vi "10-Tap 8-Bit Camera with DRAM (Host) - control.vi"() -> ()   [LabVIEW 2018]
doc: "This is the host VI for the 10-Tap 8-Bit Camera with DRAM example. This example demonstrates how to acquire images from a 10-tap, 8-bit, extended configuration, Camera Link camera and display the images on the host. This example supports area scan and line scan cameras for both continuous and finite acquisitions.\n\nThis example also demonstrates the use of DRAM as a frame buffer for very high speed acquisitions. Data packing and flow-control are also employed to maximize use of the available DRAM and FIFOs in terms of both memory space and performance.\n\nAdditionally, the example demonstrates the serial server, which allows third-party camera configuration utilities to communicate with the camera using the Camera Link serial interface while this VI is running."
uses:
  <vilib>/userdefined/High Color/nirio_resource_hc.ctl
  <vilib>/Platform/TimedLoop/XDataNode/timing_clust.ctl
  <vilib>/Platform/TimedLoop/XDataNode/nitl_modes.ctl
  <vilib>/Platform/TimedLoop/XDataNode/wakeup.ctl
  <vilib>/DAQmx/write.llb/DAQmx Write (Analog DBL 1Chan 1Samp).vi
  <vilib>/FPGAPlugInAG/PCIe-1473R/niLvFpga_Open_PCIe-1473R.vi
  <vilib>/rvi/interface/common/dynamic/niFpgaDynamicAddResources.vi
  <vilib>/FPGAPlugInAG/Dynamic/niLvFpga_Reset_Dynamic.vi
  <userlib>/DAQNavi Polymorphic VI/create/DAQNavi Create Channel(CI-UpDown Count Value).vi
  <vilib>/Utility/error.llb/Error Cluster From Error Code.vi
  <vilib>/rvi/errors/niLvFpgaAdjustHostInterfaceError.vi
  <vilib>/FPGAPlugInAG/Dynamic/niLvFpga_Run_Dynamic.vi
  <vilib>/rvi/interface/common/niFpgaWaitOnOcc.vi
  <userlib>/DAQNavi Polymorphic VI/read/DAQNavi Read (Counter Count Value 1Chan 1Samp).vi
  <vilib>/DAQmx/miscellaneous.llb/DAQmx Fill In Error Info.vi
  <vilib>/FPGAPlugInAG/Dynamic/niLvFpga_Close_Dynamic.vi
  <vilib>/platform/TimedLoop/XDataNode/XDataNode.xnode
  <vilib>/rvi/interface/nirviOpenFPGA/nirviOpenFPGA.xnode
  FPGA Bitfiles/10-Tap8-bitCamer_FPGATarget_10-Tap8-bitCamer_C490DC32.lvbitx
  <vilib>/rvi/interface/nirviMethod/nirviMethod.xnode
  <vilib>/rvi/interface/nirviReadWriteControl/nirviReadWriteControl.xnode
  <vilib>/rvi/interface/nirviCloseFPGA/nirviCloseFPGA.xnode
  <vilib>/rvi/interface/Simulation/niFpgaSimulationCallBeginRW.vi
  <vilib>/rvi/errors/niLvFpgaMergeErrorWithErrorCode.vi
  NiFpgaLv.dll
  <vilib>/FPGAPlugInAG/Dynamic/niLvFpga_ConfigureFifo_Dynamic.vi
  <vilib>/FPGAPlugInAG/Dynamic/niLvFpga_StartFifo_Dynamic.vi
  <vilib>/FPGAPlugInAG/Dynamic/niLvFpga_ReadFifo_Dynamic.vi
  <vilib>/Platform/TimedLoop/XDataNode/XDNodeRunTimeDep.lvlib
  <resource>/objmgr/ni.dex.rc
  MPC_dll_4_vs17_cv3_4/x64/Release/MPC_dll_4_vs17_cv3_4.dll
  fish tracking dll vc17 opencv3_4/x64/Release/fish tracking dll vc17 opencv3_4.dll
panel:
  in  "Templates size":i32=70
  in  "display":bool=TRUE
  out "Image":T1(plugin-control)
  in  "reset 2":bool
  in  "reset frame":bool
  in  "reset position":bool
  out "max load a frame":dbl
  out "max load a position":dbl
  out "# elements in queue":i32
  out "element":dbl[](array[numeric])
  in  "start sending":bool
  in  "Target IP Address":string="192.168.1.19"
  out "connected":bool
  in  "Acquire":bool
  in  "Frames To Acquire":u32 caption="Frames To Acquire\n(0 = infinite)"
  in  "Templates Path":path=path "F:/TrackingUsingOpenCV3_with_bkg_subtr_and_pred_and_temp_matching_nodisplay/templates"
  out "max distance 2":i32
  out "out of FOV 2":i32
  in  "count":bool
  in  "shift_head2yolk":i32=22
  out "max distance":i32
  out "out of FOV":i32
  out "Stage Position Y":i32=520
  out "Stage Position X":i32=520
  out "#timeout3":i32
  out "#timeout1":i32
  out "max time4 image loading":dbl
  out "max time3 total":dbl
  out "max time2 detection":dbl
  out "max time1 detection+command":dbl
  out "time loading a frame":dbl
  in  "gammaY":dbl=0.3 format="%#_13g"
  in  "gammaX":dbl=0.3 format="%#_13g"
  in  "predict length":i32=6
  in  "length of fish_history":i32=3
  in  "m(length of kernel)":i32=30
  out "Heading":cluster{dbl, dbl}
  in  "length_fish":i32=115
  in  "width_fish":i32=23
  out "Time out":bool
  out "BKG_Global":T1(plugin-control)
  in  "update ratio":dbl
  in  "tan(theta)":dbl=-0.0165
  in  "pixel/mm":dbl=29.9
  out "process":i32
  in  "Target Y":i32(slide)=180 min=0 max=384 scale=130.0..230.0
  in  "Target X":i32(slide)=180 min=0 max=520 scale=130.0..230.0
  out "y":dbl
  out "x":dbl
  in  "Controller":picture
  out "Y Resolution":i32
  out "X Resolution":i32
  in  "center":bool
  in  "Track":bool
  out "Frame #":i32=72
  out "电压2":dbl
  out "电压1":dbl
  in  "Bkg Image Path":path=path "F:/TrackingUsingOpenCV3_with_bkg_subtr_and_pred_and_temp_matching_nodisplay/fish tracking dll vc17 opencv3_4/bkg_global.png"
  out "fish FOUND":bool
  in  "Object Threshold":i32=84
  in  "shift":i32=14
  in  "ROI_height":i32=110
  in  "ROI_witdth":i32=110
  out "Centroid":cluster{"x":i32, "y":i32}
  out "TimeDelay":dbl
  in  "BinThreshold":i32=90
  in  "DMA Buffer Size\n(In Images)":u32=64 caption="DMA Buffer Size"
  in  "Signal Mapping":T2(ring)=enum."Basler 10-tap"
  out "Acq In Progress":bool
  in  "Line Scan":bool
  in  "Cancel":bool
  out "Acq'd Frame Width":u32
  in  "Stopped":bool
  in  "RIO Device":T3="RIO0"
  out "DMA Write Timeout":bool
  in  "Start Serial Server":bool=TRUE
  out "Frames Acq'd":u32
  out "Acq'd Frame Height":u32
  in  "Stop":bool
  in  "Image Height":u32=360 max=65535
  in  "Image Width":u32=360 max=65535 step=40
  out "Initialized":bool
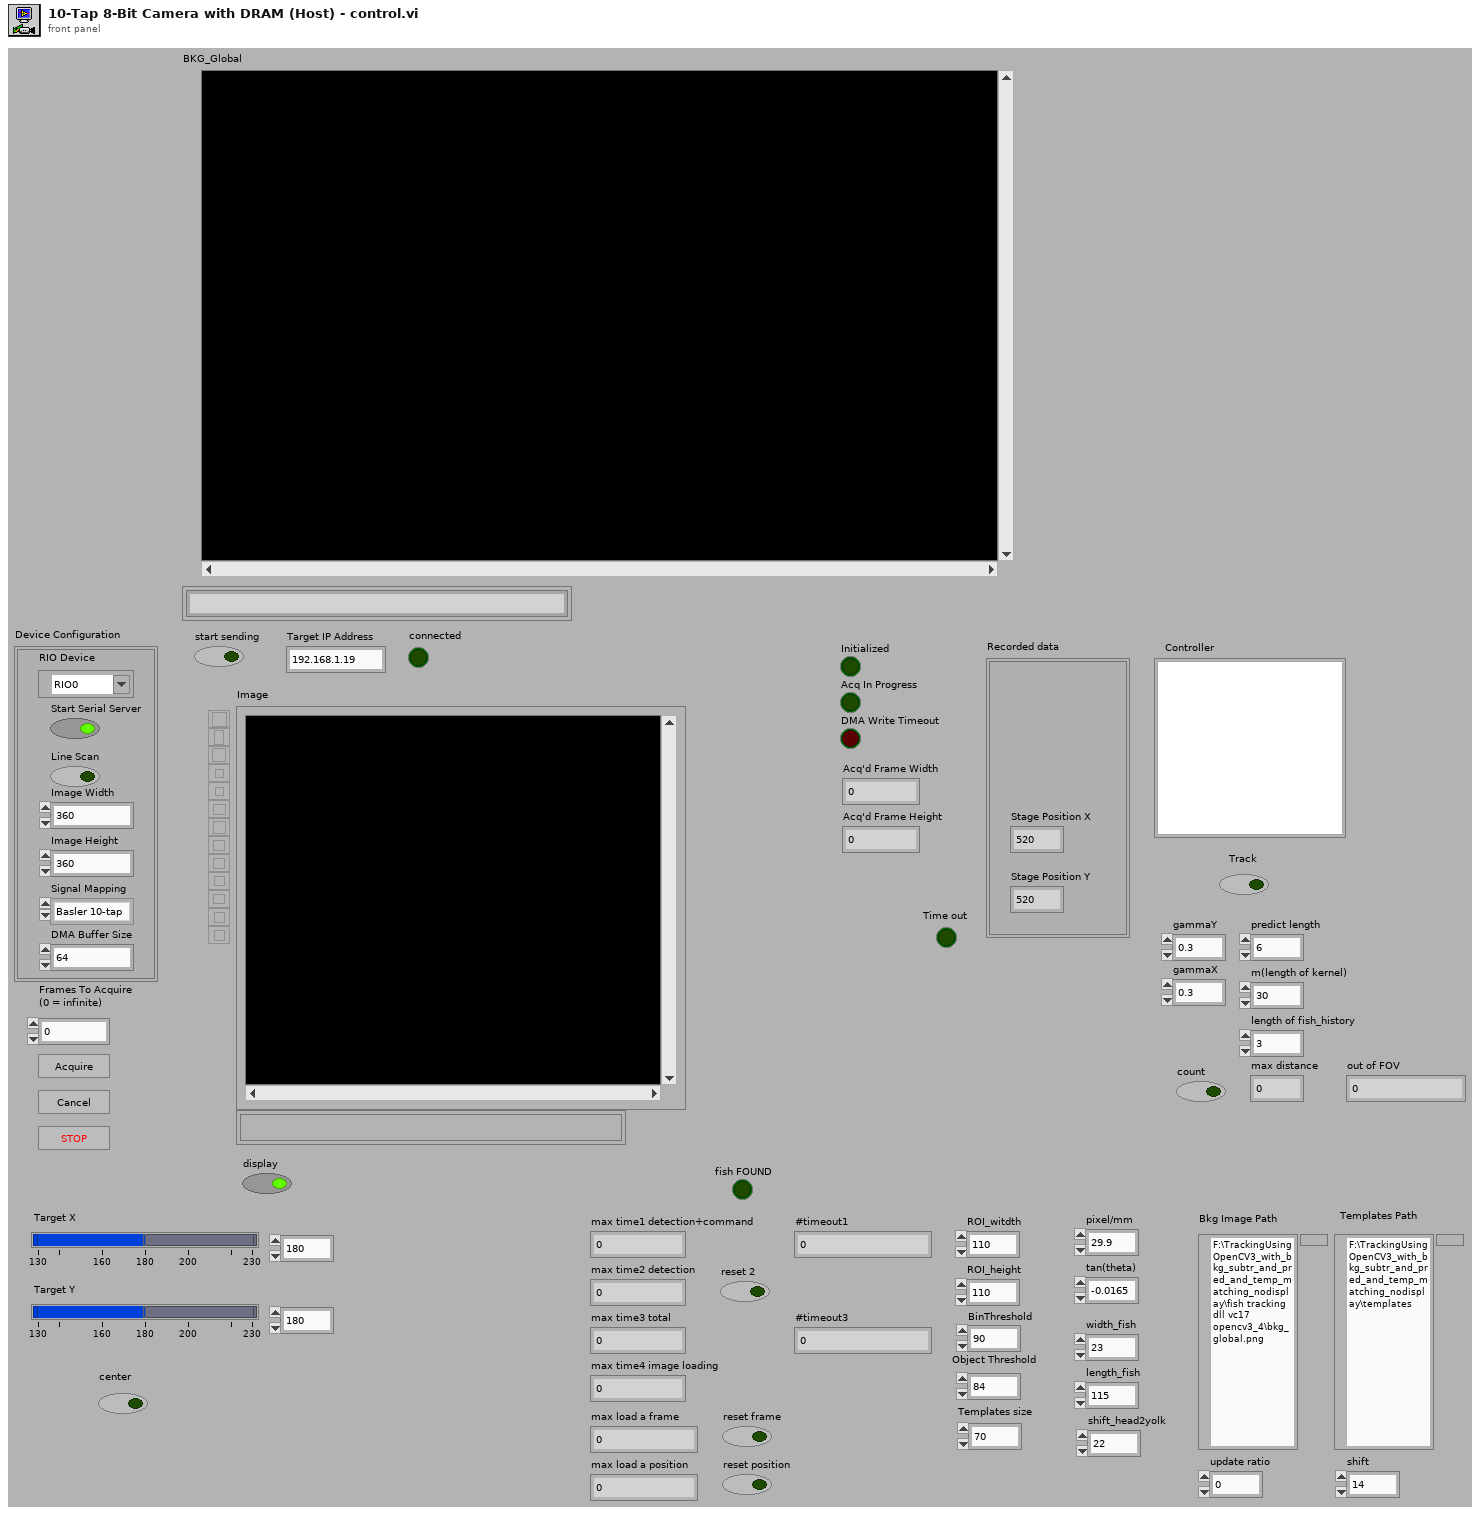
[diagram p1: front panel]
types:
  T1 = typedef "IMAQ Image.ctl" = refnum<image>
  T2 = enum8{"Standard", "Basler 10-tap", "Vosskühler 10-tap"}
  T3 = typedef "nirio_resource_hc.ctl" = tag
  T4 = typedef "Image Type" = u32
  T5 = typedef "XDNodeRunTimeDep.lvlib/timing_clust.ctl" = cluster{"Expected End [f-1]":u64, "Actual End [f-1]":u64, "Finished Late? [f-1]":bool, "Expected End [i-1]":u64, "Actual End [i-1]":u64, "Finished Late? [i-1]":bool, "Expected Start [i]":u64, "Actual Start [i]":u64, "Expected Start [f]":u64, "Actual Start [f]":u64, "Source Name":string, "Structure Name":string, "Period":i64, "Deadline":i64, "Offset":i64, "Start":i64, "Priority":i32, "Timeout":i32, "Mode":T6, "Wakeup Reason":T7, "Error":errorcluster, "Source Type":string, "Secondary Source Type":string, "Global End Time":u64, "Global Start Time":u64, "Frame Duration":u64, "Iteration Duration":u64, "Assigned CPU":i32, "I/O Scan Engine Mode":u32}
  T6 = typedef "XDNodeRunTimeDep.lvlib/nitl_modes.ctl" = enum32{"No Change", "Process missed periods, maintain original phase", "Discard missed periods, maintain original phase", "Process missed periods, ignore original phase", "Discard missed periods, ignore original phase"}
  T7 = typedef "XDNodeRunTimeDep.lvlib/wakeup.ctl" = enum32{"Normal", "Aborted", "Asynchronous wakeup", "Timing source error", "Timed loop error", "Timeout"}
  T8 = enum16{"big-endian, network order", "native, host order", "little-endian"}
  T9 = enum32{"Map Pixel Pointer", "Unmap Pixel Pointer", "Get Pixels Infos"}
  T10 = typedef "LVPoint32TypeDef.ctl" = cluster{"Horizontal":i32, "Vertical":i32}
  T11 = typedef "LVPositionTypeDef.ctl" = cluster{"Left":i32, "Top":i32}
  T12 = typedef "LVBoundsTypeDef.ctl" = cluster{"Width":u32, "Height":u32}
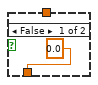
[diagram p6: hidden frame]
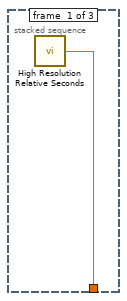
[diagram p7: hidden frame]
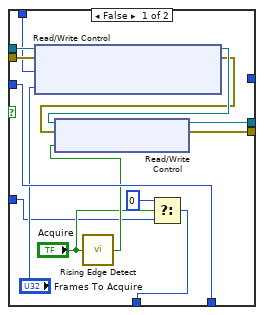
[diagram p8: hidden frame]
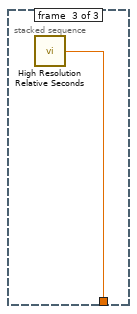
[diagram p9: hidden frame]
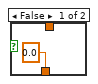
[diagram p10: hidden frame]
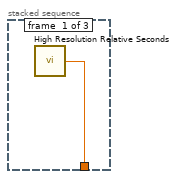
[diagram p11: hidden frame]
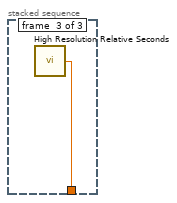
[diagram p12: hidden frame]
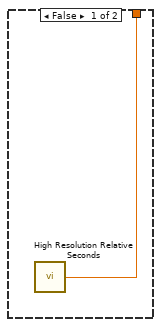
[diagram p18: hidden frame]
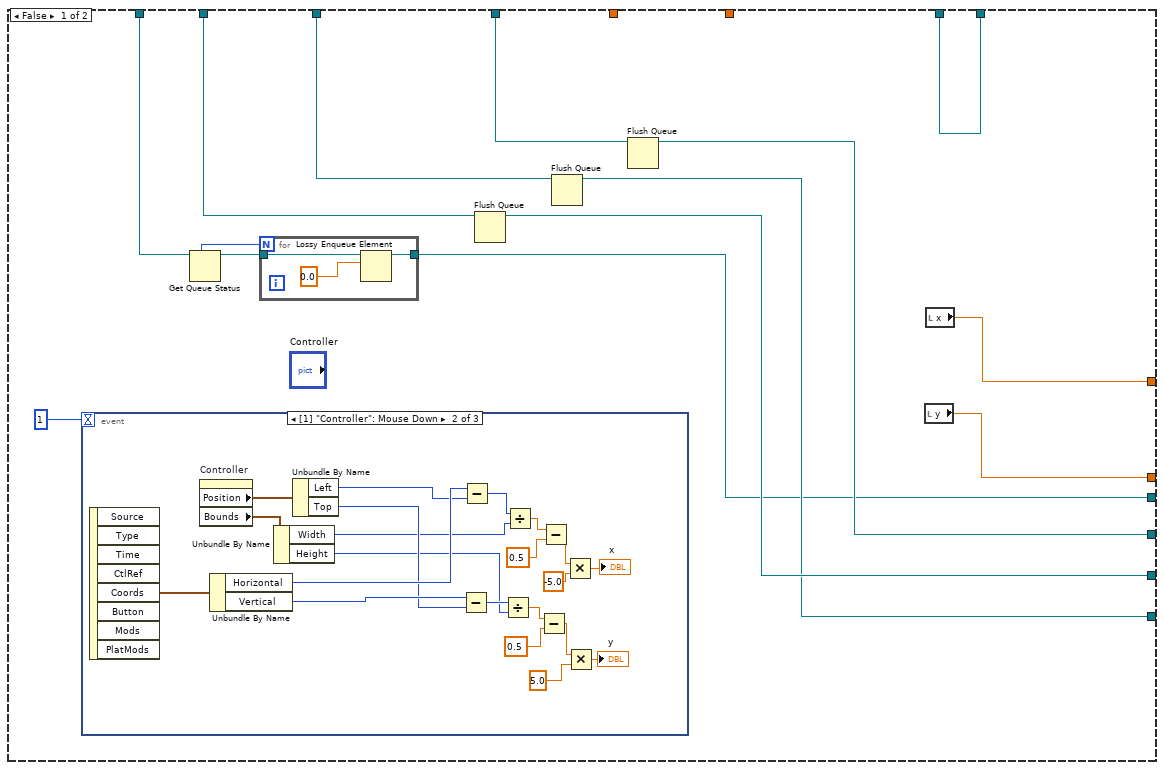
[diagram p20: hidden frame]
diagram:
  w33 = 72 ("n_templates")
  w35 = 0
  w56 = 2
  w50 = 0
  w57 = 0.0
  w82 = T4 0 items=["Grayscale (U8)", "Grayscale (I16)", "Grayscale (SGL)", "Complex (CSG)", "RGB (U32)", "HSL (U32)", "RGB (U64)", "Grayscale (U16)"] ("Image Type")
  w96 = refnum<k21> "Stage_Y"  # DAQmx任务名
  w97 = refnum<k21> "Stage_X"  # DAQmx任务名
  w99 = T4 0 items=["Grayscale (U8)", "Grayscale (I16)", "Grayscale (SGL)", "Complex (CSG)", "RGB (U32)", "HSL (U32)", "RGB (U64)", "Grayscale (U16)"] ("Image Type")
  w105 = u32 8  # Pixels per DMA word
  w139 = T4 0 items=["Grayscale (U8)", "Grayscale (I16)", "Grayscale (SGL)", "Complex (CSG)", "RGB (U32)", "HSL (U32)", "RGB (U64)", "Grayscale (U16)"] ("Image Type")
  # "If your camera outputs active-low enable\nsignals or does not use DVAL then you \ncan change the configuration here."
  # "Configure the DMA FIFO memory buffer to be\nlarge enough for several frames. This provides\nbuffering to help deal with system latencies."
  # "Start running\nthe FPGA VI."
  # "Reset FPGA to clear\nany current state."
  # "Read the specified image\nwidth and height. In this\nexample, these must be set\nbefore starting the VI."
  # "Merge any errors.\nClean up the image.\nClose the FPGA reference.\nDisplay any errors."
  # "Acquire frames as requested.\nUse the width and height to determine how much data to read from the DMA FIFO.\nConvert the data into a Vision Image for display."
  # "Monitor the acquisition status"
  # "Start the Serial Server to allow serial communication\nwith the camera. This allows third-party camera\nconfiguration utilites to be used."
  # "Create an image of the type to be displayed."
  # "Initialize the acquisition interface on the FPGA.  This will\nwait until a pixel clock is detected from the camera."
  # "Initialize the DMA FIFO for transferring\ndata from FPGA target to the host."
  # "Configure the Camera Link interface.\nThis needs to be done prior to running\nthe FPGA block diagram."
  # "Open a reference to the FPGA bitstream\nand initialize the user interface."
  n1 = flat-sequence {
    tunnel: [w145] -> w132
    tunnel: [w144] -> w143
    frame #0 {
      w148 = u32 0 ("Num Lines Acq'd")
      w147 = FALSE ("stop")
      n2 = local write "DMA Write Timeout"(w147) -> ()
      n3 = local write "Acq'd Frame Width"(w148) -> ()
      n4 = local write "Acq'd Frame Height"(w148) -> ()
      n5 = local write "Stopped"(w147) -> ()
      n6 = local write "Frames Acq'd"(w148) -> ()
      n7 = local write "Initialized"(w147) -> ()
      n8 = xnode "打开FPGA VI引用句柄"("resource name"="RIO Device") -> ("FPGA VI Reference Out"=w145:refnum<k20>, "error out"=w144:errorcluster)  [unwired: 1 in]
    }
  }
  n9 = xnode "Invoke Method"("FPGA VI Reference In"=w132, "error in"=w143) -> ("FPGA VI Reference Out"=w122:refnum<k20>, "error out"=w124:errorcluster)
  n10 = xnode "Read/Write Control"("FPGA VI Reference In"=w122, "error in"=w124, "CL Config.FVAL Active High"=TRUE ("IO Module Config.CL FVAL Active High"), "CL Config.LVAL Active High"=TRUE ("IO Module Config.CL LVAL Active High"), "CL Config.DVAL Active High"=TRUE ("IO Module Config.CL DVAL Active High"), "CL Config.Spare Active High"=TRUE ("IO Module Config.CL Spare Active High"), "CL Config.Line Scan"="Line Scan", "Acq Control.Ignore DVAL"=FALSE ("CL Config.Line Scan"), "CL Config.Configuration"=enum8{"Base", "Medium", "Full"}."Full", "CL Config.Signal Mapping"="Signal Mapping") -> ("FPGA VI Reference Out"=w125:refnum<k20>, "error out"=w123:errorcluster)
  n11 = xnode "Invoke Method"("FPGA VI Reference In"=w125, "error in"=w123) -> ("FPGA VI Reference Out"=w102:refnum<k20>, "error out"=w101:errorcluster)  [unwired: 1 in]
  n12 = Multiply(x="Image Height", y="Image Width") -> (x*y=w104:u32)
  n13 = Quotient & Remainder(x=w104, y=w105) -> (floor(x/y)=w103:u32)  [unwired: 1 out]
  n14 = Multiply(x=w103, y="DMA Buffer Size\n(In Images)") -> (x*y=w116:u32)
  n15 = xnode "Invoke Method"("FPGA VI Reference In"=w102, "error in"=w101, "请求的深度"=w116) -> ("FPGA VI Reference Out"=w131:refnum<k20>, "error out"=w130:errorcluster)  [unwired: 1 out]
  n16 = xnode "Invoke Method"("FPGA VI Reference In"=w131, "error in"=w130) -> ("FPGA VI Reference Out"=w117:refnum<k20>, "error out"=w129:errorcluster)
  n17 = xnode "读取/写入控件"("FPGA VI Reference In"=w117, "error in"=w129, "Acq Control.Initialize"=TRUE ("Arm Acquisition")) -> ("FPGA VI Reference Out"=w142:refnum<k20>, "error out"=w141:errorcluster)
  n18 = while {
    tunnel: w142 -> [w156]
    tunnel: w141 -> [w155]
    tunnel: [w154] -> w113
    tunnel: [w158] -> w112
    i -> [w150]
    stop <- w161 stop-if-true
    # "A custom error is generated if the acquisition unit has not become\ninitialized within 2 seconds. This typically occurs when a camera is\nnot connected, is not powered, or is not of the correct type."
    n19 = xnode "读取/写入控件"("FPGA VI Reference In"=w156, "error in"=w155) -> ("FPGA VI Reference Out"=w154:refnum<k20>, "error out"=w153:errorcluster, "Acq Status.Initialized"=w152:bool)
    n20 = Wait (ms)(milliseconds to wait=u32 100) -> ()  [unwired: 1 out]
    n21 = Greater?(x=w150, y=20) -> (0:w151:bool)
    n22 = case shown="True" w151 {
      tunnel: [w163 FALSE] -> w157
      tunnel: w152 -> [w163 _]
      tunnel: w153 -> [w162 w165]
      tunnel: [w162 w167] -> w158
      frame False {
      }
      frame True {
        n23 = Merge Errors(w165, errorcluster {"status"=TRUE, "code"=-8999, "source"="Acquisition Initialization: This error typically occurs when a camera is not properly connected, is not powered, or is not of the correct type."} ("error in")) -> (w167:errorcluster)
      }
    }
    "Initialized" <- w157
    n24 = Unbundle By Name(w158) -> ("status"=w160:bool)
    n25 = Or(x=w160, y=w157) -> (x .or. y?=w161:bool)
  }
  n26 = case shown="True" "Start Serial Server" {
    tunnel: [_ w168] -> w133
    tunnel: w113 -> [_ w169]
    frame False {
    }
    frame True {
      n27 = control-ref of="Stopped"() -> (w170:refnum<vi>)
      n28 = call "SerialServer.vi"("Stop Refnum"=w170, "FPGA VI Reference In"=w169) -> ("FPGA VI Reference Out"=w168:refnum<k20>)  [unwired: 5 in]
    }
  }
  n29 = call "IMAQ Create"("Image Name"="Image", "Image Type"=w139, "error in (no error)"=w112) -> ("New Image"=w109:T1, "error out"=w108:errorcluster)  [unwired: 2 in]
  n30 = Concatenate Strings("//" ("reader url"), "Target IP Address") -> (w17:string)
  n31 = Concatenate Strings(w17, "/reader1" ("reader url")) -> (w15:string)
  n32 = Create Network Stream Writer Endpoint(7:70, 9:0.0, 10:w15, 11:"writer") -> (0:w20:errorcluster, 3:w22:refnum<k21>)  [unwired: 3 in]
  n33 = property class="Network Stream Endpoint"(reference=w22, error in=w20) -> (reference out=w9:refnum<k21>, error out=w8:errorcluster, "Connected"=→"connected":bool)
  n34 = Add(x="length of fish_history", y=1) -> (x+y=w52:i32)
  n35 = Initialize Array(0.0, 7) -> (w12:dbl[])
  n36 = Obtain Queue(max queue size (-1, unlimited)=3, name (unnamed)="tracking result" ("Image Name"), element data type=w12) -> (queue out=w10:refnum<queue>)  [unwired: 2 in, 2 out]
  n37 = Multiply(x=w56, y=w52) -> (x*y=w49:i32)
  n38 = To Unsigned Byte Integer(number=w35) -> (unsigned 8bit integer=w36:u8)
  n39 = Initialize Array(w36, w35, w35, w35) -> (w34:u8[][][])
  n40 = node-c288() -> (w7:T5)  [unwired: 4 in]
  n41 = for {
    N: w33 -> [_]
    shift-right: [w172] -> w32
    shift-left: w34 -> [w173]
    i -> [w171]
    w177 = T4 0 items=["Grayscale (U8)", "Grayscale (I16)", "Grayscale (SGL)", "Complex (CSG)", "RGB (U32)", "HSL (U32)", "RGB (U64)", "Grayscale (U16)"] ("Image Type")
    n42 = Number To Decimal String(number=w171) -> (decimal integer string=w181:string)  [unwired: 1 in]
    n43 = Concatenate Strings(w181, ".jpg") -> (w180:string)
    n44 = Build Path(base path="Templates Path", name or relative path=w180) -> (appended path=w179:path)
    n45 = call "IMAQ Create"("Image Name"="Temp", "Image Type"=w177) -> ("New Image"=w176:T1)  [unwired: 3 in, 1 out]
    n46 = call "IMAQ ReadFile"("File Path"=w179, "Image"=w176) -> ("Image Out"=w175:T1)  [unwired: 5 in, 4 out]
    n47 = call "IMAQ ImageToArray"("Image"=w175) -> ("Image Pixels (U8)"=w174:u8[][])  [unwired: 3 in, 4 out]
    n48 = Insert Into Array(array=w173, index (dim 0)=w171, new element=w174) -> (w172:u8[][][])  [unwired: 2 in]
  }
  n49 = Add(x="m(length of kernel)", y=1) -> (x+y=w37:i32)
  n50 = timed-loop {
    tunnel: w10 -> [w190]
    tunnel: w9 -> [w189]
    tunnel: w8 -> [w188]
    tunnel: [w187] -> w3
    tunnel: [w186] -> w2
    tunnel: [w185] -> w1
    timing: w7 -> [_]
    timing-out: [_] -> w6
    stop <- w184 stop-if-true
    n51 = node-c288() -> ()  [unwired: 1 in, 1 out]
    n52 = case shown="True" "start sending" {
      tunnel: w189 -> [w195 w208]
      tunnel: w188 -> [w194 w207]
      tunnel: w190 -> [w196 w198]
      tunnel: [w196 w206] -> w187
      tunnel: [w195 w201] -> w186
      tunnel: [w194 w200] -> w185
      frame False {
      }
      frame True {
        w202 = 0
        n53 = Get Queue Status(queue=w198) -> (queue out=w199:refnum<queue>, # elements in queue=w197:i32)  [unwired: 2 in, 6 out]
        n54 = disable-structure shown="Disabled" {
          disable-tunnel: w197 -> [w209 _]
          frame Disabled {
            "# elements in queue" <- w209
          }
          frame Enabled {
          }
        }
        n55 = Dequeue Element(queue=w199) -> (queue out=w206:refnum<queue>, element=w205:dbl[])  [unwired: 2 in, 2 out]
        n56 = disable-structure shown="Disabled" {
          disable-tunnel: w205 -> [w210 _]
          frame Disabled {
            "element" <- w210
          }
          frame Enabled {
          }
        }
        n57 = shared-variable-write(w208, w207, w205, w202) -> (w204:refnum<k21>, w203:errorcluster)  [unwired: 1 out]
        n58 = Flush Stream(8:w203, 9:w202, 11:w204) -> (0:w200:errorcluster, 3:w201:refnum<k21>)  [unwired: 1 in, 1 out]
      }
    }
    n59 = local read "Stop"() -> (w184:bool)
    n60 = node-c288() -> ()  [unwired: 1 in, 1 out]
  }
  n61 = Multiply(x=w56, y=w37) -> (x*y=w55:i32)
  n62 = Obtain Queue(max queue size (-1, unlimited)=w55, name (unnamed)="command_history", element data type=w57) -> (queue out=w59:refnum<queue>)  [unwired: 2 in, 2 out]
  n63 = Obtain Queue(max queue size (-1, unlimited)=w49, name (unnamed)="stage_position_history", element data type=w50) -> (queue out=w48:refnum<queue>)  [unwired: 2 in, 2 out]
  n64 = Obtain Queue(max queue size (-1, unlimited)=w49, name (unnamed)="fish_tr_history", element data type=w50) -> (queue out=w61:refnum<queue>)  [unwired: 2 in, 2 out]
  n65 = Obtain Queue(max queue size (-1, unlimited)=w49, name (unnamed)="fish_heading_history", element data type=w57) -> (queue out=w60:refnum<queue>)  [unwired: 2 in, 2 out]
  n66 = for "For循环" {
    N: w55 -> [_]
    tunnel: w59 -> [w213]
    tunnel: [w212] -> w58
    n67 = Lossy Enqueue Element(queue=w213, element=0.0) -> (queue out=w212:refnum<queue>)  [unwired: 1 in, 3 out]
  }
  n68 = call-poly <userlib>:"DAQNavi Create Channel.vi"("physical channels"="PCI-1784,BID#1/cntr0" ("Image Name"), "signal counting type"="AbPhaseX4" ("Image Name"), "initial value"="0" ("Image Name")) -> ("task out"=w76:i32)  [unwired: 11 in, 1 out]
  n69 = call-poly <userlib>:"DAQNavi Create Channel.vi"("physical channels"="PCI-1784,BID#1/cntr1" ("Image Name"), "signal counting type"="AbPhaseX4" ("Image Name"), "initial value"="0" ("Image Name")) -> ("task out"=w75:i32)  [unwired: 11 in, 1 out]
  n70 = call "IMAQ Create"("Image Name"="BkgImageOpenCV", "Image Type"=w82) -> ("New Image"=w84:T1)  [unwired: 3 in, 1 out]
  n71 = node-c288() -> (w27:T5)  [unwired: 4 in]
  n72 = call <userlib>:"DAQNavi Start Task.vi"("task in"=w76) -> ("task out"=w72:i32)  [unwired: 9 in, 1 out]
  n73 = call <userlib>:"DAQNavi Start Task.vi"("task in"=w75) -> ("task out"=w71:i32)  [unwired: 9 in, 1 out]
  n74 = call "IMAQ Create"("Image Name"="DstImageOpenCV", "Image Type"=w99) -> ("New Image"=w98:T1)  [unwired: 3 in, 1 out]
  n75 = call "IMAQ ReadFile"("File Path"="Bkg Image Path", "Image"=w84) -> ("Image Out"=w81:T1)  [unwired: 5 in, 4 out]
  n76 = while {
    tunnel: w113 -> [w224]
    tunnel: [w227] -> w126
    stop <- w226 stop-if-true
    w217 = u32 10  # Pixels per clock
    # "Update status indicators"
    n77 = Wait Until Next ms Multiple(millisecond multiple=u32 100) -> ()  [unwired: 1 out]
    n78 = xnode "Read/Write Control"("FPGA VI Reference In"=w224) -> ("error out"=w223:errorcluster, "Acq Status.Lines Per Frame"=→"Acq'd Frame Height":u32, "Acq Status.Frames Acq'd"=→"Frames Acq'd":u32, "Acq Status.Clocks Per Line"=w218:u32, "Acq Status.Acq In Progress"=→"Acq In Progress":bool, "Acq Status.DMA Write Timeout"=w215:bool)  [unwired: 1 in, 1 out]
    "DMA Write Timeout" <- w215
    n79 = Multiply(x=w218, y=w217) -> (x*y=→"Acq'd Frame Width":u32)
    n80 = local read "Stopped"() -> (w214:bool)
    n81 = Compound Arithmetic op=AND(w215, invert w214) -> (w216:bool)
    n82 = case shown="True" w216 {
      tunnel: w223 -> [w232 _]
      tunnel: [w232 errorcluster {"status"=TRUE, "code"=-8999, "source"="DMA Write Timeout: The write operation to the DMA FIFO on the FPGA timed out. This can be caused by the DMA FIFO not being started or the DMA FIFO overflowing. Make sure that Start is being called on the DMA FIFO. Also make sure that the host application is reading from the DMA FIFO fast enough to prevent it from overflowing."} ("error out")] -> w227
      frame False {
      }
      frame True {
      }
    }
    n83 = flat-sequence {
      tunnel: w227 -> [w231]
      tunnel: [w229] -> w226
      frame #0 {
        n84 = Unbundle By Name(w231) -> ("status"=w230:bool)
        n85 = Or(x=w230, y="Stopped") -> (x .or. y?=w229:bool)
        n86 = local write "Stopped"(w229) -> ()
      }
    }
  }
  n87 = node-c288(w6) -> ()  [unwired: 1 out]
  n88 = Release Queue(queue=w3) -> ()  [unwired: 2 in, 3 out]
  n89 = Flush Stream(8:w1, 11:w2) -> (0:w4:errorcluster, 3:w5:refnum<k21>)  [unwired: 2 in, 1 out]
  n90 = Destroy Stream Endpoint(8:w4, 11:w5) -> ()  [unwired: 1 out]
  n91 = Open/Create/Replace File(file path (use dialog)=path "E:/Time.txt" ("Folder"), operation (0:open)=4) -> (refnum out=w41:refnum<file>)  [unwired: 4 in, 2 out]
  n92 = call <vilib>:"DAQmx Start Task.vi"("task/channels in"=w96) -> ("task out"=w94:refnum<k21>)  [unwired: 13 in, 1 out]
  n93 = call <vilib>:"DAQmx Start Task.vi"("task/channels in"=w97) -> ("task out"=w95:refnum<k21>)  [unwired: 13 in, 1 out]
  n94 = timed-loop {
    tunnel: w113 -> [w351]
    tunnel: w108 -> [w350]
    tunnel: w103 -> [w247]
    tunnel: "Image Height" -> [w246]
    tunnel: "Image Width" -> [w355]
    tunnel: w109 -> [w354]
    tunnel: [w236] -> w127
    tunnel: [w353] -> w138
    tunnel: [w352] -> w135
    tunnel: w98 -> [w349]
    tunnel: w95 -> [w348]
    tunnel: w94 -> [w347]
    tunnel: [w346] -> w93
    tunnel: [w345] -> w92
    tunnel: w81 -> [w344]
    tunnel: w72 -> [w337]
    tunnel: w71 -> [w336]
    tunnel: [w335] -> w68
    tunnel: [w334] -> w67
    shift-right: [w340] -> _
    shift-left: u32 0 -> [w341]
    shift-right: [w338] -> _
    shift-left: cluster{"y":i32, "x":i32} {"y"=0, "x"=0} ("Centroid") -> [w339]
    tunnel: w58 -> [w333]
    tunnel: w61 -> [w332]
    tunnel: w60 -> [w331]
    tunnel: w48 -> [w330]
    tunnel: [w329] -> w47
    tunnel: [w328] -> w46
    tunnel: [w327] -> w45
    tunnel: [w326] -> w44
    tunnel: w41 -> [w324]
    tunnel: [w323] -> w40
    shift-right: [w322] -> _
    shift-left: _ -> [w321]
    tunnel: w33 -> [w320]
    tunnel: w32 -> [w319]
    tunnel: w10 -> [w318]
    timing: w27 -> [_]
    timing-out: [_] -> w26
    border: u32 0 -> [_]
    i -> [w325]
    stop <- w342 stop-if-true
    # "Read one frame\nfrom DMA FIFO"
    # "If we're in an acquisition, wait until\nwe have at least one frame to read."
    n95 = node-c288() -> ()  [unwired: 1 in, 1 out]
    n96 = stacked-sequence {
      tunnel: [_ w366 _] -> w353
      tunnel: w351 -> [_ w365 _]
      tunnel: w350 -> [_ w364 _]
      tunnel: [_ w363 _] -> w236
      tunnel: [_ w362 _] -> w317
      tunnel: w247 -> [_ w361 _]
      tunnel: w246 -> [_ w360 _]
      tunnel: [w359 _ _] -> w244
      tunnel: [_ _ w414] -> w245
      frame #0 {
        n97 = call <vilib>:"High Resolution Relative Seconds.vi"() -> ("relative seconds"=w359:dbl)
      }
      frame #1 {
        n98 = while {
          tunnel: [w372] -> w362
          tunnel: w361 -> [w369]
          shift-right: [w380] -> w366
          shift-left: w365 -> [w379]
          shift-right: [w373] -> w363
          shift-left: w364 -> [w378]
          tunnel: w360 -> [w367]
          stop <- w368 stop-if-true
          n99 = feedback #1() -> (w374:u32)
          n100 = while {
            tunnel: w379 -> [w410]
            tunnel: w378 -> [w409]
            tunnel: [w407] -> w377
            tunnel: [w408] -> w376
            tunnel: w374 -> [w413]
            tunnel: [w411] -> w370
            stop <- w412 stop-if-true
            n101 = xnode "Read/Write Control"("FPGA VI Reference In"=w410, "error in"=w409, "Acq Control.Cancel Acq"="Cancel") -> ("FPGA VI Reference Out"=w408:refnum<k20>, "error out"=w407:errorcluster, "Acq Status.Acq In Progress"=w406:bool, "Acq Status.Frames Acq'd"=w405:u32)
            n102 = Greater?(x=w405, y=w413) -> (0:w411:bool)
            n103 = Compound Arithmetic op=OR(invert w406, w411) -> (w412:bool)
          }
          n104 = case shown="True" w370 {
            tunnel: w369 -> [w392 w403]
            tunnel: [w387 w402] -> w380
            tunnel: w377 -> [w394 w401]
            tunnel: w376 -> [w393 w400]
            tunnel: [w381 w399] -> w375
            tunnel: w374 -> [w382 w398]
            tunnel: [w386 w397] -> w373
            tunnel: [_ w396] -> w372
            tunnel: [w392 w395] -> w371
            tunnel: w367 -> [w391 _]
            frame False {
              n105 = xnode "Read/Write Control"("FPGA VI Reference In"=w393, "error in"=w394, "Acq Control.Line Scan Height"=w391, "Acq Control.Frames To Acq"="Frames To Acquire") -> ("FPGA VI Reference Out"=w389:refnum<k20>, "error out"=w388:errorcluster)
              n106 = call "Rising Edge Detect.vi"("Input"="Acquire") -> ("Pulse"=w385:bool)  [unwired: 4 in]
              n107 = xnode "Read/Write Control"("FPGA VI Reference In"=w389, "error in"=w388, "Acq Control.Acquire"=w385) -> ("FPGA VI Reference Out"=w387:refnum<k20>, "error out"=w386:errorcluster)
              n108 = Select(t=u32 0, s="Acquire", f=w382) -> (s? t:f=w381:u32)
            }
            frame True {
              n109 = xnode "Invoke Method"("FPGA VI Reference In"=w400, "error in"=w401, "元素数量"=w403) -> ("FPGA VI Reference Out"=w402:refnum<k20>, "error out"=w397:errorcluster, "数据"=w396:u64[], "剩余元素"=w395:u32)  [unwired: 1 in]
              n110 = Increment(x=w398) -> (x+1=w399:u32)
            }
          }
          n111 = feedback-in #1(w375) -> ()
          n112 = Less?(x=w371, y=w369) -> (x < y?=w368:bool)
        }
      }
      frame #2 {
        n113 = call <vilib>:"High Resolution Relative Seconds.vi"() -> ("relative seconds"=w414:dbl)
      }
    }
    n114 = disable-structure shown="Disabled" {
      disable-tunnel: w325 -> [w356 _]
      frame Disabled {
        "process" <- w356
      }
      frame Enabled {
      }
    }
    n115 = Not(x="reset frame") -> (.not. x?=w235:bool)
    n116 = Boolean To (0,1)(Boolean=w235) -> (0, 1=w240:i16)
    n117 = Subtract(x=w245, y=w244) -> (x-y=w241:dbl)
    n118 = feedback #2(-inf) -> (w243:dbl)
    n119 = Max & Min(x=w241, y=w243) -> (max(x,y)=w238:dbl)  [unwired: 1 out]
    n120 = Multiply(x=w238, y=w240) -> (x*y=w237:dbl)
    n121 = feedback-in #2(w237) -> ()
    n122 = case shown="True" w235 {
      tunnel: w238 -> [_ w358]
      tunnel: [0.0 w358] -> w234
      frame False {
      }
      frame True {
      }
    }
    "max load a frame" <- w234
    n123 = flat-sequence {
      tunnel: w321 -> [w434]
      tunnel: w330 -> [w435]
      tunnel: w331 -> [w436]
      tunnel: w332 -> [w437]
      tunnel: w333 -> [w438]
      tunnel: w336 -> [w432]
      tunnel: w337 -> [w433]
      tunnel: w339 -> [w439]
      tunnel: w341 -> [w440]
      tunnel: w344 -> [w441]
      tunnel: w349 -> [w442]
      tunnel: w317 -> [w443]
      tunnel: w354 -> [w444]
      tunnel: w355 -> [w445]
      tunnel: w246 -> [w446]
      tunnel: [w446] -> w316
      tunnel: [w445] -> w315
      tunnel: [w444] -> w314
      tunnel: [w443] -> w313
      tunnel: [w442] -> w312
      tunnel: [w441] -> w311
      tunnel: [w440] -> w310
      tunnel: [w439] -> w309
      tunnel: [w438] -> w308
      tunnel: [w437] -> w307
      tunnel: [w436] -> w306
      tunnel: [w435] -> w305
      tunnel: [w434] -> w304
      tunnel: [w431] -> w303
      tunnel: [w430] -> w302
      tunnel: [w429] -> w301
      tunnel: [w428] -> w300
      tunnel: w320 -> [w428]
      tunnel: [w427] -> w299
      tunnel: w319 -> [w427]
      tunnel: w318 -> [w426]
      tunnel: [w426] -> w298
      tunnel: [w489] -> w297
      tunnel: [w488] -> w296
      tunnel: [w487] -> w295
      tunnel: [w486] -> w294
      tunnel: [w485] -> w293
      tunnel: [w484] -> w292
      tunnel: [w483] -> w291
      tunnel: [w482] -> w290
      tunnel: [w464] -> w289
      tunnel: [w462] -> w288
      tunnel: [w481] -> w287
      tunnel: [w480] -> w286
      tunnel: [w479] -> w285
      tunnel: [w478] -> w284
      tunnel: [w474] -> w283
      tunnel: [w463] -> w282
      tunnel: w316 -> [w489]
      tunnel: w315 -> [w488]
      tunnel: w314 -> [w487]
      tunnel: w313 -> [w486]
      tunnel: w312 -> [w485]
      tunnel: w311 -> [w484]
      tunnel: w310 -> [w483]
      tunnel: w309 -> [w482]
      tunnel: w308 -> [w481]
      tunnel: w307 -> [w480]
      tunnel: w306 -> [w479]
      tunnel: w305 -> [w478]
      tunnel: w304 -> [w472]
      tunnel: w303 -> [w464]
      tunnel: w302 -> [w463]
      tunnel: w301 -> [w462]
      tunnel: [w461] -> w281
      tunnel: w300 -> [w461]
      tunnel: [w460] -> w280
      tunnel: w299 -> [w460]
      tunnel: [w459] -> w279
      tunnel: w298 -> [w459]
      tunnel: w325 -> [w525]
      tunnel: w324 -> [w524]
      tunnel: [w523] -> w323
      tunnel: w297 -> [w575]
      tunnel: w296 -> [w574]
      tunnel: w295 -> [w573]
      tunnel: w294 -> [w571]
      tunnel: w293 -> [w494]
      tunnel: w292 -> [w545]
      tunnel: w291 -> [w542]
      tunnel: w290 -> [w492]
      tunnel: w289 -> [w518]
      tunnel: w288 -> [w517]
      tunnel: w287 -> [w536]
      tunnel: w286 -> [w535]
      tunnel: w285 -> [w534]
      tunnel: w284 -> [w533]
      tunnel: w283 -> [w521]
      tunnel: [w495] -> w278
      tunnel: [w541] -> w277
      tunnel: [w518] -> w276
      tunnel: [w517] -> w275
      tunnel: [w504] -> w274
      tunnel: [w532] -> w273
      tunnel: [w531] -> w272
      tunnel: [w530] -> w271
      tunnel: [w529] -> w270
      tunnel: [w520] -> w269
      tunnel: [w519] -> w268
      tunnel: w282 -> [w505]
      tunnel: w281 -> [w515]
      tunnel: w280 -> [w513]
      tunnel: w279 -> [w508]
      tunnel: w278 -> [w826]
      tunnel: [w826] -> w267
      tunnel: w277 -> [w825]
      tunnel: [w825] -> w266
      tunnel: w276 -> [w824]
      tunnel: [w824] -> w265
      tunnel: w275 -> [w823]
      tunnel: [w823] -> w264
      tunnel: w274 -> [w822]
      tunnel: [w822] -> w263
      tunnel: w273 -> [w821]
      tunnel: [w821] -> w262
      tunnel: w272 -> [w820]
      tunnel: [w820] -> w261
      tunnel: w271 -> [w819]
      tunnel: [w819] -> w260
      tunnel: w270 -> [w818]
      tunnel: [w818] -> w259
      tunnel: w269 -> [w817]
      tunnel: [w817] -> w258
      tunnel: w268 -> [w816]
      tunnel: [w816] -> w257
      tunnel: w267 -> [w842]
      tunnel: w266 -> [w841]
      tunnel: w265 -> [w840]
      tunnel: w264 -> [w839]
      tunnel: w263 -> [w838]
      tunnel: w262 -> [w837]
      tunnel: w261 -> [w836]
      tunnel: w260 -> [w835]
      tunnel: w259 -> [w834]
      tunnel: [w833] -> w345
      tunnel: [w832] -> w346
      tunnel: w348 -> [w831]
      tunnel: w347 -> [w830]
      tunnel: w258 -> [w829]
      tunnel: w257 -> [w828]
      tunnel: [w842] -> w256
      tunnel: [w841] -> w255
      tunnel: [w840] -> w254
      tunnel: [w839] -> w253
      tunnel: [w838] -> w252
      tunnel: [w837] -> w251
      tunnel: [w836] -> w250
      tunnel: [w835] -> w249
      tunnel: [w834] -> w248
      tunnel: [w844] -> w326
      tunnel: [w845] -> w327
      tunnel: [w846] -> w328
      tunnel: [w847] -> w329
      tunnel: [w848] -> w338
      tunnel: [w849] -> w334
      tunnel: [w850] -> w335
      tunnel: [w851] -> w340
      tunnel: [w852] -> w352
      tunnel: w256 -> [w852]
      tunnel: w255 -> [w851]
      tunnel: w254 -> [w850]
      tunnel: w253 -> [w849]
      tunnel: w252 -> [w848]
      tunnel: w251 -> [w847]
      tunnel: w250 -> [w846]
      tunnel: w249 -> [w845]
      tunnel: w248 -> [w844]
      tunnel: [w843] -> w322
      frame #0 {
        n124 = stacked-sequence {
          tunnel: w433 -> [_ w456 _]
          tunnel: w432 -> [_ w455 _]
          tunnel: [_ w454 _] -> w431
          tunnel: [_ w453 _] -> w430
          tunnel: [_ w452 _] -> w429
          tunnel: [w449 _ _] -> w425
          tunnel: [_ _ w458] -> w424
          frame #0 {
            n125 = call <vilib>:"High Resolution Relative Seconds.vi"() -> ("relative seconds"=w449:dbl)
          }
          frame #1 {
            n126 = call-poly <userlib>:"DAQNavi Read.vi"("task in"=w455) -> ("data"=w451:i32, "task out"=w452:i32)  [unwired: 9 in]
            n127 = call-poly <userlib>:"DAQNavi Read.vi"("task in"=w456) -> ("data"=w457:i32, "task out"=w454:i32)  [unwired: 9 in]
            "Stage Position X" <- w457
            n128 = Negate(x=w451) -> (-x=w450:i32)
            "Stage Position Y" <- w450
            n129 = Bundle("data"=w457, w450) -> (w453:cluster{"data":i32, i32})  [unwired: 1 in]
          }
          frame #2 {
            n130 = call <vilib>:"High Resolution Relative Seconds.vi"() -> ("relative seconds"=w458:dbl)
          }
        }
        n131 = Not(x="reset position") -> (.not. x?=w417:bool)
        n132 = Boolean To (0,1)(Boolean=w417) -> (0, 1=w419:i16)
        n133 = Subtract(x=w424, y=w425) -> (x-y=w421:dbl)
        n134 = feedback #3(-inf) -> (w423:dbl)
        n135 = Max & Min(x=w421, y=w423) -> (max(x,y)=w416:dbl)  [unwired: 1 out]
        n136 = Multiply(x=w416, y=w419) -> (x*y=w418:dbl)
        n137 = feedback-in #3(w418) -> ()
        n138 = case shown="True" w417 {
          tunnel: w416 -> [_ w448]
          tunnel: [0.0 w448] -> w415
          frame False {
          }
          frame True {
          }
        }
        "max load a position" <- w415
      }
      frame #1 {
        n139 = call <vilib>:"High Resolution Relative Seconds.vi"() -> ("relative seconds"=w474:dbl)
        n140 = feedback #4() -> (w475:dbl)  [unwired: 1 in]
        n141 = feedback-in #4(w474) -> ()
        n142 = Subtract(x=w474, y=w475) -> (x-y=w477:dbl)
        n143 = disable-structure shown="Disabled" {
          disable-tunnel: w477 -> [w490 _]
          frame Disabled {
            "TimeDelay" <- w490
          }
          frame Enabled {
          }
        }
        n144 = Greater?(x=w477, y=0.0045) -> (0:w469:bool)
        "Time out" <- w469
        n145 = Subtract(x=w474, y=w472) -> (x-y=w473:dbl)
        n146 = disable-structure shown="Disabled" {
          disable-tunnel: w473 -> [w491 _]
          frame Disabled {
            "time loading a frame" <- w491
          }
          frame Enabled {
          }
        }
        n147 = Select(t=1, s=w469, f=0) -> (s? t:f=w466:i32)
        n148 = feedback #5(0) -> (w467:i32)
        n149 = Add(x=w466, y=w467) -> (x+y=w465:i32)
        "#timeout3" <- w465
        n150 = feedback-in #5(w465) -> ()
      }
      frame #2 {
        w537 = 0.0
        w556 = T9."Map Pixel Pointer" ("Function")
        # "Convert U64 array\nto U8 array"
        # "Convert array to\nimage for display"
        n151 = Add(x=1, y=w542) -> (x+y=w541:u32)
        n152 = Flatten To String(anything=w571, prepend array or string size? (T)=FALSE, byte order (0:big-endian, network order)=T8."native, host order") -> (data string=w569:string)  [unwired: 1 in, 2 out]
        n153 = disable-structure shown="Disabled" {
          disable-tunnel: w541 -> [w576 _]
          frame Disabled {
            "Frame #" <- w576
          }
          frame Enabled {
          }
        }
        n154 = String To Byte Array(string=w569) -> (unsigned byte array=w568:u8[])
        n155 = call "IMAQ GetImageSize"("Image"=w545) -> ("Y Resolution"=w543:i32, "X Resolution"=w544:i32)  [unwired: 3 in, 1 out]
        n156 = Reshape Array(w568, w575, w574) -> (w572:u8[][])
        n157 = call "IMAQ ArrayToImage"("Image Pixels (U8)"=w572, "Image"=w573) -> ("Image Out"=w495:T1)  [unwired: 8 in, 1 out]
        n158 = call "IMAQ GetImagePixelPtr"("Function"=w556, "Image"=w545) -> ("LineWidth(Pixels)"=w558:i32, "Pixel Pointer out"=w559:u64)  [unwired: 4 in, 4 out]
        n159 = expression code="atan(x)"("tan(theta)") -> (w547:dbl)
        n160 = Divide(x="pixel/mm", y=10000.0) -> (x/y=w550:dbl)
        n161 = Divide(x="pixel/mm", y=12800.0) -> (x/y=w549:dbl)
        n162 = call "IMAQ GetImageSize"("Image"=w495) -> ("Y Resolution"=w509:i32, "X Resolution"=w510:i32)  [unwired: 3 in, 1 out]
        "X Resolution" <- w510
        "Y Resolution" <- w509
        n163 = call "IMAQ GetImagePixelPtr"("Function"=w556, "Image"=w495) -> ("LineWidth(Pixels)"=w563:i32, "Pixel Pointer out"=w567:u64)  [unwired: 4 in, 4 out]
        n164 = call "IMAQ SetImageSize"("Y Resolution"=w509, "X Resolution"=w510, "Image"=w494) -> ("Image Out"=w507:T1)  [unwired: 2 in, 1 out]
        n165 = Bundle(w537, w537) -> (w512:cluster{dbl, dbl})  [unwired: 1 in]
        n166 = call "IMAQ GetImagePixelPtr"("Function"=w556, "Image"=w507) -> ("LineWidth(Pixels)"=w565:i32, "Pixel Pointer out"=w566:u64)  [unwired: 4 in, 4 out]
        n167 = dll-call lib="F:/TrackingUsingOpenCV3_with_bkg_subtr_and_pred_and_temp_matching_nodisplay - 20190402/fish tracking dll vc17 opencv3_4/x64/Release/fish tracking dll vc17 opencv3_4.dll" fn="?find_centroid@@YAHPEADH0H0HHHHHPEAEHHPEAV?$Point_@H@cv@@NNNHHHHHHH22PEAV?$Point_@N@2@N@Z"("ImagePtrSrc"=w567, "LineWidthSrc"=w563, "ImagePtrDst"=w566, "LineWidthDst"=w565, "ImagePtrBkg"=w559, "LineWidthBkg"=w558, "Width"=w510, "Height"=w509, "BkgWidth"=w544, "BkgHeight"=w543, "templates"=w513, "n_templates"=w515, "TemplatesSize"="Templates size", "position"=w505, "scale_x"=w550, "scale_y"=w549, "theta"=w547, "BinThreshold"="BinThreshold", "counting_threshold"="Object Threshold", "ROI_witdth"="ROI_witdth", "ROI_height"="ROI_height", "width_fish"="width_fish", "length_fish"="length_fish", "shift"="shift", "centroid_in"=w492, "Centroid"=w492, "heading_vector"=w512, "Update_Ratio_Bkg"="update ratio") -> ("return type"=w540:i32, "Centroid"=w504:cluster{"y":i32, "x":i32}, "heading_vector"=w503:cluster{dbl, dbl})  [unwired: 29 in, 2 out]
        n168 = Quotient & Remainder(x=w525, y=2) -> (x-y*floor(x/y)=w527:i32)  [unwired: 1 out]
        n169 = Equal To 0?(x=w540) -> (x = 0?=w511:bool)
        "fish FOUND" <- w511
        n170 = disable-structure shown="Disabled" {
          disable-tunnel: w503 -> [w577 _]
          frame Disabled {
            "Heading" <- w577
          }
          frame Enabled {
          }
        }
        n171 = disable-structure shown="Disabled" {
          disable-tunnel: w504 -> [w578 _]
          frame Disabled {
            "Centroid" <- w578
          }
          frame Enabled {
          }
        }
        n172 = Equal?(x=w527, y=0) -> (x = y?=w506:bool)
        n173 = Unbundle(w505) -> ("data"=w502:i32, w501:i32)
        n174 = Unbundle(w503) -> (w499:dbl, w500:dbl)
        n175 = Unbundle(w504) -> ("y"=w498:i32, "x"=w497:i32)
        n176 = Build Array(w502, w501, w498, w497, w499, w500) -> (w496:dbl[])
        n177 = case shown="True" w506 {
          tunnel: [w579 w583] -> w522
          tunnel: w508 -> [_ w585]
          tunnel: w496 -> [_ w584]
          tunnel: w494 -> [_ w581]
          frame False {
            n178 = call <vilib>:"High Resolution Relative Seconds.vi"() -> ("relative seconds"=w579:dbl)
          }
          frame True {
            n179 = call <vilib>:"High Resolution Relative Seconds.vi"() -> ("relative seconds"=w583:dbl)
            n180 = Build Array (concatenate)(w583, w584) -> (w582:dbl[])
            n181 = case shown="True" "display" {
              tunnel: w581 -> [_ w586]
              frame False {
              }
              frame True {
                "Image" <- w586
              }
            }
            n182 = Lossy Enqueue Element(queue=w585, element=w582) -> ()  [unwired: 1 in, 4 out]
          }
        }
        n183 = And(x=w511, y="Track") -> (x .and. y?=w493:bool)
        n184 = case shown="True" w493 {
          tunnel: [w598 w654] -> w520
          tunnel: [w599 w655] -> w519
          tunnel: w536 -> [w589 w723]
          tunnel: w535 -> [w596 w722]
          tunnel: w534 -> [w594 w721]
          tunnel: w498 -> [_ w640]
          tunnel: w497 -> [_ w641]
          tunnel: w499 -> [_ w713]
          tunnel: w500 -> [_ w712]
          tunnel: w533 -> [w592 w706]
          tunnel: w502 -> [_ w704]
          tunnel: w501 -> [_ w703]
          tunnel: [w590 w680] -> w532
          tunnel: [w591 w685] -> w531
          tunnel: [w595 w684] -> w530
          tunnel: [w593 w683] -> w529
          tunnel: w521 -> [_ w660]
          tunnel: w524 -> [w597 w659]
          tunnel: [w597 w658] -> w523
          tunnel: w522 -> [_ w656]
          frame False {
            n185 = event shown="[1] \"Controller\": Mouse Down" {
              selector: _ -> [_ _ _]
              dyn-events: _ -> [_ _ _]
              timeout: 1 -> [_ _ _]
              event "Controller": Mouse Up {
                n186 = event-data() -> ()  [unwired: 1 in, 8 out]
                n187 = local write "x"(0.0) -> ()
                n188 = local write "y"(0.0) -> ()
              }
              event "Controller": Mouse Down {
                n189 = event-data() -> ("Coords"=w626:T10)  [unwired: 1 in, 7 out]
                n190 = property on="Controller" class="Pict"() -> ("Position"=w625:T11, "Bounds"=w620:T12)  [unwired: 2 in, 2 out]
                n191 = Unbundle By Name(w626) -> ("Horizontal"=w624:i32, "Vertical"=w622:i32)
                n192 = Unbundle By Name(w620) -> ("Width"=w618:u32, "Height"=w614:u32)
                n193 = Unbundle By Name(w625) -> ("Left"=w623:i32, "Top"=w621:i32)
                n194 = Subtract(x=w622, y=w621) -> (x-y=w615:i32)
                n195 = Subtract(x=w624, y=w623) -> (x-y=w619:i32)
                n196 = Divide(x=w615, y=w614) -> (x/y=w607:dbl)
                n197 = Divide(x=w619, y=w618) -> (x/y=w617:dbl)
                n198 = Subtract(x=w607, y=0.5) -> (x-y=w610:dbl)
                n199 = Subtract(x=w617, y=0.5) -> (x-y=w611:dbl)
                n200 = Multiply(x=w611, y=-5.0) -> (x*y=→"x":dbl)
                n201 = Multiply(x=w610, y=5.0) -> (x*y=→"y":dbl)
              }
              event Timeout {
                n202 = event-data() -> ()  [unwired: 1 in, 3 out]
              }
            }
            n203 = Get Queue Status(queue=w589) -> (queue out=w588:refnum<queue>, max queue size=w587:i32)  [unwired: 2 in, 6 out]
            n204 = for "For循环" {
              N: w587 -> [_]
              tunnel: w588 -> [w603]
              tunnel: [w602] -> w590
              n205 = Lossy Enqueue Element(queue=w603, element=0.0) -> (queue out=w602:refnum<queue>)  [unwired: 1 in, 3 out]
            }
            n206 = Flush Queue(queue=w596) -> (queue out=w595:refnum<queue>)  [unwired: 1 in, 2 out]
            n207 = Flush Queue(queue=w594) -> (queue out=w593:refnum<queue>)  [unwired: 1 in, 2 out]
            n208 = Flush Queue(queue=w592) -> (queue out=w591:refnum<queue>)  [unwired: 1 in, 2 out]
            n209 = local read "y"() -> (w599:dbl)
            n210 = local read "x"() -> (w598:dbl)
          }
          frame True {
            w645 = 0
            w652 = 23
            w665 = 0.0
            w674 = 2
            w678 = TRUE
            w690 = 1.0
            n211 = local read "Target Y"() -> (w642:i32)
            n212 = case shown="False" "center" {
              tunnel: ["Target X" 509] -> w663
              tunnel: ["Target Y" 384] -> w662
              frame False {
              }
              frame True {
              }
            }
            n213 = Subtract(x=w641, y=w642) -> (x-y=w636:i32)
            n214 = Absolute Value(x=w636) -> (abs(x)=w635:i32)
            n215 = Bundle("Target X"=w663, "Target Y"=w662) -> (w661:cluster{"Target X":i32, "Target Y":i32})  [unwired: 1 in]
            n216 = Greater?(x=w635, y=w652) -> (0:w650:bool)
            n217 = local read "Target X"() -> (w639:i32)
            n218 = Get Queue Status(queue=w723, return elements? (F)=w678) -> (queue out=w681:refnum<queue>, elements=w669:dbl[])  [unwired: 1 in, 6 out]
            n219 = Subtract(x=w640, y=w639) -> (x-y=w634:i32)
            n220 = Get Queue Status(queue=w722) -> (queue out=w717:refnum<queue>, max queue size=w672:i32, # elements in queue=w718:i32)  [unwired: 2 in, 5 out]
            n221 = Equal?(x=w718, y=0) -> (x = y?=w719:bool)
            n222 = Absolute Value(x=w634) -> (abs(x)=w633:i32)
            n223 = Quotient & Remainder(x=w672, y=2) -> (floor(x/y)=w670:i32)  [unwired: 1 out]
            n224 = case shown="True" w719 {
              tunnel: w717 -> [w801 w804]
              tunnel: w640 -> [w800 w805]
              tunnel: w670 -> [_ w806]
              tunnel: [w797 w803] -> w716
              tunnel: w641 -> [w799 w802]
              frame False {
                n225 = Lossy Enqueue Element(queue=w801, element=w800) -> (queue out=w798:refnum<queue>)  [unwired: 1 in, 3 out]
                n226 = Lossy Enqueue Element(queue=w798, element=w799) -> (queue out=w797:refnum<queue>)  [unwired: 1 in, 3 out]
              }
              frame True {
                n227 = for "For循环" {
                  N: w806 -> [_]
                  tunnel: w805 -> [w811]
                  tunnel: w804 -> [w810]
                  tunnel: [w807] -> w803
                  tunnel: w802 -> [w808]
                  n228 = Lossy Enqueue Element(queue=w810, element=w811) -> (queue out=w809:refnum<queue>)  [unwired: 1 in, 3 out]
                  n229 = Lossy Enqueue Element(queue=w809, element=w808) -> (queue out=w807:refnum<queue>)  [unwired: 1 in, 3 out]
                }
              }
            }
            n230 = Get Queue Status(queue=w716, return elements? (F)=w678) -> (queue out=w684:refnum<queue>, elements=w679:i32[])  [unwired: 1 in, 6 out]
            n231 = Greater?(x=w633, y=w652) -> (0:w651:bool)
            n232 = Or(x=w650, y=w651) -> (x .or. y?=w649:bool)
            n233 = Get Queue Status(queue=w721) -> (queue out=w710:refnum<queue>, max queue size=w675:i32, # elements in queue=w714:i32)  [unwired: 2 in, 5 out]
            n234 = Equal?(x=w714, y=0) -> (x = y?=w711:bool)
            n235 = Select(t=1, s=w649, f=w645) -> (s? t:f=w647:i32)
            n236 = local read "tan(theta)"() -> (w692:dbl)
            n237 = local read "pixel/mm"() -> (w695:dbl)
            n238 = Quotient & Remainder(x=w675, y=w674) -> (floor(x/y)=w673:i32)  [unwired: 1 out]
            n239 = case shown="True" w711 {
              tunnel: w710 -> [w786 w789]
              tunnel: w713 -> [w785 w790]
              tunnel: w673 -> [_ w791]
              tunnel: [w782 w788] -> w709
              tunnel: w712 -> [w784 w787]
              frame False {
                n240 = Lossy Enqueue Element(queue=w786, element=w785) -> (queue out=w783:refnum<queue>)  [unwired: 1 in, 3 out]
                n241 = Lossy Enqueue Element(queue=w783, element=w784) -> (queue out=w782:refnum<queue>)  [unwired: 1 in, 3 out]
              }
              frame True {
                n242 = for "For循环" {
                  N: w791 -> [_]
                  tunnel: w790 -> [w796]
                  tunnel: w789 -> [w795]
                  tunnel: [w793] -> w788
                  tunnel: w787 -> [w792]
                  n243 = Lossy Enqueue Element(queue=w795, element=w796) -> (queue out=w794:refnum<queue>)  [unwired: 1 in, 3 out]
                  n244 = Lossy Enqueue Element(queue=w794, element=w792) -> (queue out=w793:refnum<queue>)  [unwired: 1 in, 3 out]
                }
              }
            }
            n245 = Get Queue Status(queue=w709, return elements? (F)=w678) -> (queue out=w683:refnum<queue>, elements=w667:dbl[])  [unwired: 1 in, 6 out]
            n246 = local read "m(length of kernel)"() -> (w701:i32)
            n247 = local read "length of fish_history"() -> (w699:i32)
            n248 = feedback #6(w645) -> (w631:i32)
            n249 = expression code="atan(x)"(w692) -> (w691:dbl)
            n250 = Divide(x=1.0, y=w695) -> (x/y=w693:dbl)
            n251 = Get Queue Status(queue=w706) -> (queue out=w705:refnum<queue>, max queue size=w677:i32, # elements in queue=w707:i32)  [unwired: 2 in, 5 out]
            n252 = Quotient & Remainder(x=w677, y=w674) -> (floor(x/y)=w676:i32)  [unwired: 1 out]
            n253 = Equal?(x=w707, y=0) -> (x = y?=w657:bool)
            n254 = case shown="True" w657 {
              tunnel: w705 -> [w771 w774]
              tunnel: w704 -> [w770 w775]
              tunnel: w676 -> [_ w776]
              tunnel: [w767 w773] -> w702
              tunnel: w703 -> [w769 w772]
              frame False {
                n255 = Lossy Enqueue Element(queue=w771, element=w770) -> (queue out=w768:refnum<queue>)  [unwired: 1 in, 3 out]
                n256 = Lossy Enqueue Element(queue=w768, element=w769) -> (queue out=w767:refnum<queue>)  [unwired: 1 in, 3 out]
              }
              frame True {
                n257 = for "For循环" {
                  N: w776 -> [_]
                  tunnel: w775 -> [w781]
                  tunnel: w774 -> [w780]
                  tunnel: [w777] -> w773
                  tunnel: w772 -> [w778]
                  n258 = Lossy Enqueue Element(queue=w780, element=w781) -> (queue out=w779:refnum<queue>)  [unwired: 1 in, 3 out]
                  n259 = Lossy Enqueue Element(queue=w779, element=w778) -> (queue out=w777:refnum<queue>)  [unwired: 1 in, 3 out]
                }
              }
            }
            n260 = Get Queue Status(queue=w702, return elements? (F)=w678) -> (queue out=w685:refnum<queue>, elements=w668:i32[])  [unwired: 1 in, 6 out]
            n261 = Max & Min(x=w633, y=w635) -> (max(x,y)=w644:i32)  [unwired: 1 out]
            n262 = Divide(x=w690, y=10000.0) -> (x/y=w687:dbl)
            n263 = Divide(x=w690, y=12800.0) -> (x/y=w686:dbl)
            n264 = feedback #7(w645) -> (w637:i32)
            n265 = case shown="True" "count" {
              tunnel: [w725 w727] -> w638
              tunnel: w637 -> [_ w726]
              tunnel: w631 -> [_ w727]
              tunnel: [w725 w726] -> w630
              frame False {
                w725 = 0
                "out of FOV 2" <- w725
                "max distance 2" <- w725
              }
              frame True {
                "out of FOV" <- w727
                "max distance" <- w726
              }
            }
            n266 = Add(x=w638, y=w647) -> (x+y=w646:i32)
            n267 = feedback-in #6(w646) -> ()
            n268 = Max & Min(x=w644, y=w630) -> (max(x,y)=w643:i32)  [unwired: 1 out]
            n269 = feedback-in #7(w643) -> ()
            n270 = Bundle(w665, w665) -> (w664:cluster{dbl, dbl})  [unwired: 1 in]
            n271 = dll-call lib="F:/TrackingUsingOpenCV3_with_bkg_subtr_and_pred_and_temp_matching_nodisplay - 20190402/MPC_dll_4_vs17_cv3_4/x64/Release/MPC_dll_4_vs17_cv3_4.dll" fn="?MPC_dll@@YAHHHHNNNHNNNNNPEAV?$Point_@H@cv@@PEANPEAH21PEAV?$Point_@N@2@@Z"("m"=w701, "predict_length"="predict length", "fish_history_length"=w699, "gammaX"="gammaX", "gammaY"="gammaY", "max_command"=10.0, "shift_head2yolk"="shift_head2yolk", "scale_x"=w693, "scale_y"=w693, "theta"=w691, "scale_x2"=w687, "scale_y2"=w686, "dst_fish_position"=w661, "command_history_array"=w669, "position_history_array"=w668, "fish_tr_history_c_array"=w679, "fish_direction_history_c_array"=w667, "c0"=w664) -> ("return type"=w629:i32, "c0"=w666:cluster{dbl, dbl})  [unwired: 20 in, 2 out]
            n272 = Equal To 0?(x=w629) -> (x = 0?=w627:bool)
            n273 = Not(x=w627) -> (.not. x?=w628:bool)
            n274 = case shown="False" w628 {
              tunnel: w660 -> [w754 w766]
              tunnel: w659 -> [w753 w765]
              tunnel: [w753 w764] -> w658
              tunnel: w656 -> [w755 w763]
              frame False {
                w743 = -inf
                n275 = local read "time loading a frame"() -> (w746:dbl)
                n276 = local read "TimeDelay"() -> (w748:dbl)
                n277 = call <vilib>:"High Resolution Relative Seconds.vi"() -> ("relative seconds"=w756:dbl)
                n278 = Not(x="reset 2") -> (.not. x?=w732:bool)
                n279 = Boolean To (0,1)(Boolean=w732) -> (0, 1=w731:i16)
                n280 = Subtract(x=w756, y=w754) -> (x-y=w733:dbl)
                n281 = Subtract(x=w755, y=w754) -> (x-y=w750:dbl)
                n282 = feedback #8(w743) -> (w752:dbl)
                n283 = feedback #9(w743) -> (w749:dbl)
                n284 = feedback #10(w743) -> (w751:dbl)
                n285 = Max & Min(x=w733, y=w752) -> (max(x,y)=w742:dbl)  [unwired: 1 out]
                "max time1 detection+command" <- w742
                n286 = feedback-in #8(w742) -> ()
                n287 = Max & Min(x=w748, y=w749) -> (max(x,y)=w745:dbl)  [unwired: 1 out]
                "max time3 total" <- w745
                n288 = feedback-in #9(w745) -> ()
                n289 = Max & Min(x=w750, y=w751) -> (max(x,y)=w730:dbl)  [unwired: 1 out]
                "max time2 detection" <- w730
                n290 = Multiply(x=w730, y=w731) -> (x*y=w729:dbl)
                n291 = feedback-in #10(w729) -> ()
                n292 = Greater?(x=w733, y=0.003) -> (0:w740:bool)
                n293 = feedback #11(w743) -> (w747:dbl)
                n294 = Select(t=1, s=w740, f=0) -> (s? t:f=w737:i32)
                n295 = Max & Min(x=w746, y=w747) -> (max(x,y)=w744:dbl)  [unwired: 1 out]
                "max time4 image loading" <- w744
                n296 = feedback-in #11(w744) -> ()
                n297 = feedback #12(0) -> (w736:i32)
                n298 = Add(x=w737, y=w736) -> (x+y=w735:i32)
                "#timeout1" <- w735
                n299 = feedback-in #12(w735) -> ()
              }
              frame True {
                n300 = call <vilib>:"High Resolution Relative Seconds.vi"() -> ("relative seconds"=w762:dbl)
                n301 = local read "TimeDelay"() -> (w760:dbl)
                n302 = local read "time loading a frame"() -> (w757:dbl)
                n303 = Subtract(x=w762, y=w766) -> (x-y=w761:dbl)
                n304 = Subtract(x=w763, y=w766) -> (x-y=w759:dbl)
                n305 = Format Into String(initial string=w765, w761, w759, w760, w757, "\r") -> (resulting string=w764:refnum<file>)  [unwired: 2 in, 1 out]
              }
            }
            n306 = Unbundle(w666) -> (w654:dbl, w655:dbl)
            n307 = Lossy Enqueue Element(queue=w681, element=w654) -> (queue out=w682:refnum<queue>)  [unwired: 1 in, 3 out]
            n308 = Lossy Enqueue Element(queue=w682, element=w655) -> (queue out=w680:refnum<queue>)  [unwired: 1 in, 3 out]
          }
        }
        "BKG_Global" <- w545
      }
      frame #3 {
      }
      frame #4 {
        n309 = Negate(x=w828) -> (-x=w827:dbl)
        "电压2" <- w827
        n310 = call-poly <vilib>:"DAQmx Write.vi"("task/channels in"=w831, "data"=w829) -> ("task out"=w832:refnum<k21>)  [unwired: 11 in, 2 out]
        n311 = call-poly <vilib>:"DAQmx Write.vi"("task/channels in"=w830, "data"=w827) -> ("task out"=w833:refnum<k21>)  [unwired: 11 in, 2 out]
        "电压1" <- w829
      }
      frame #5 {
        n312 = call <vilib>:"High Resolution Relative Seconds.vi"() -> ("relative seconds"=w843:dbl)
      }
    }
    n313 = flat-sequence {
      tunnel: w236 -> [w857]
      tunnel: [w855] -> w343
      frame #0 {
        n314 = Unbundle By Name(w857) -> ("status"=w858:bool)
        n315 = local read "Stopped"() -> (w856:bool)
        n316 = Compound Arithmetic op=OR(w858, "Stop", w856) -> (w855:bool)
        n317 = local write "Stopped"(w855) -> ()
      }
    }
    n318 = feedback-in #13(w343) -> ()
    n319 = feedback #13() -> (w342:bool)  [unwired: 1 in]
    n320 = node-c288() -> ()  [unwired: 1 in, 1 out]
  }
  n321 = Close File(refnum=w40) -> ()  [unwired: 1 in, 2 out]
  n322 = call-poly <vilib>:"DAQmx Write.vi"("task/channels in"=w93, "data"=0.0) -> ("task out"=w91:refnum<k21>)  [unwired: 11 in, 2 out]
  n323 = call <vilib>:"DAQmx Stop Task.vi"("task/channels in"=w91) -> ("task out"=w87:refnum<k21>)  [unwired: 13 in, 1 out]
  n324 = call-poly <vilib>:"DAQmx Write.vi"("task/channels in"=w92, "data"=0.0) -> ("task out"=w89:refnum<k21>)  [unwired: 11 in, 2 out]
  n325 = call <vilib>:"DAQmx Stop Task.vi"("task/channels in"=w89) -> ("task out"=w86:refnum<k21>)  [unwired: 13 in, 1 out]
  n326 = call <vilib>:"DAQmx Clear Task.vi"("task in"=w87) -> ()  [unwired: 14 in, 1 out]
  n327 = call <vilib>:"DAQmx Clear Task.vi"("task in"=w86) -> ()  [unwired: 14 in, 1 out]
  n328 = node-c288(w26) -> ()  [unwired: 1 out]
  n329 = Release Queue(queue=w47) -> ()  [unwired: 2 in, 3 out]
  n330 = Release Queue(queue=w46) -> ()  [unwired: 2 in, 3 out]
  n331 = Release Queue(queue=w45) -> ()  [unwired: 2 in, 3 out]
  n332 = Release Queue(queue=w44) -> ()  [unwired: 2 in, 3 out]
  n333 = call <userlib>:"DAQNavi Stop Task.vi"("task in"=w68) -> ("task out"=w70:i32)  [unwired: 1 in, 1 out]
  n334 = Merge Errors(w127, w126) -> (w128:errorcluster)
  n335 = call <userlib>:"DAQNavi Stop Task.vi"("task in"=w67) -> ("task out"=w69:i32)  [unwired: 1 in, 1 out]
  n336 = flat-sequence {
    tunnel: w128 -> [w861]
    tunnel: [w861] -> w137
    tunnel: w135 -> [w862]
    tunnel: w133 -> [_]
    frame #0 {
      n337 = local write "Initialized"(FALSE ("Module Enabled")) -> ()
      n338 = call "IMAQ Dispose"("Image"=w862) -> ()  [unwired: 5 in, 1 out]
    }
  }
  n339 = call <userlib>:"DAQNavi Clear Task.vi"("task in"=w70) -> ()  [unwired: 2 in, 1 out]
  n340 = call <userlib>:"DAQNavi Clear Task.vi"("task in"=w69) -> ()  [unwired: 2 in, 1 out]
  n341 = xnode "关闭FPGA VI引用"("FPGA VI引用输入"=w138, "错误输入"=w137) -> ("错误输出"=w134:errorcluster)
  n342 = call <vilib>:"Simple Error Handler.vi"("error in (no error)"=w134) -> ()  [unwired: 4 in, 5 out]
